vi "MotionProfileController.vi"() -> ()   [LabVIEW 2018]
panel:
  out "MP File Ready":bool
  in  "MP CSV File Name":string
  in  "Reset MP":bool
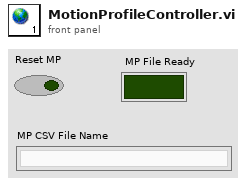
[diagram p1: front panel]
diagram:
